vi "1296_usbUart.vi"(0 "VISA resource name":refnum<visa-resource-name>, 5 "command":string, 7 "r/w":enum16{"read", "write"}(ring), 9 "resetValues":bool, 11 "error in (no error)":errorcluster) -> (4 "byte Array":string[](array[string]), 6 "byte[4]":string, 8 "byte[5]":string, 15 "error out":errorcluster)   [LabVIEW 2018]
uses:
  <vilib>/Instr/_visa.llb/VISA Flush IO Buffer Mask.ctl
  <vilib>/Instr/_visa.llb/VISA Configure Serial Port (Instr).vi
panel:
  out "write buffer":string
  out "binary[7]":string
  out "number[7]":u32
  out "byte[7]":string
  out "number[4]":u32
  out "number[5]":u32
  out "number[6]":u32
  out "binary[6]":string
  out "byte[6]":string
  out "binary[5]":string
  out "binary[4]":string
  out "binary[3]":string
  out "number[3]":u32
  out "byte[3]":string
  out "number[0]":u32
  out "number[1]":u32
  out "number[2]":u32
  out "binary[2]":string
  out "byte[2]":string
  out "binary[1]":string
  out "byte[1]":string
  out "byte[0]":string
  out "binary[0]":string
  out "valid byte":string
  out "bytes at port":u32
  out "byte count":u32
  out "read buffer":string
  # "1. set visa\n2. set r/w\n3. enter command:\naddress/command/and any data if writing.\nwrite example: 0900 0001\nread example: 0900"
  # "Read Packet:\t\t\t\t\t\t\t\t\t\t\t                                                                                                                                                                                                                                                                                                                                              Example for w/r of relay1:\t\t\t\t\t\t\t\t\t\t\t\t\t\t\nAddress\t0x01 - Speed\t0x02 - Distance\t0x03 - Resistance\t0x04 - Incline\t0x09 - Box Control\t\t\t\t\t\t                                                                                                                                                                                                                0x09\tRead relay1\t\t\t\t\t\t\t\t\t\t\t\t\t\nCommand\tcommand for each protocol above - to be determined\t\t\t\t\t\t\t\t\t\t                                                                                                                                                                                                                                                   0x00\t\t\t\t\t\t\t\t\t\t\t\t\t\t\nType\t0x03 - Read\t0x06 - Write\t\t\t\t\t\t\t\t\t                                                                                                                                                                                                                                                                                                                    0x03\t\t\t\t\t\t\t\t\t\t\t\t\t\t\nByte Count\t0x01 would = Two bytes of data\t\t\t\t\t\t\t\t\t\t                                                                                                                                                                                                                                                                                          0x02\t\t\t\t\t\t\t\t\t\t\t\t\t\t\nEnd Charactors\t0x0D0A\t\t\t\t\t\t\t\t\t\t                                                                                                                                                                                                                                                                                                                             0x0D0A\t\t\t\t\t\t\t\t\t\t\t\t\t\t\n\t\t\t\t\t\t\t\t\t\t\t\t\t\t\t\t\t\t\t\t\t\t\t\t\t\n\t\t\t\t\t\t\t\t\t\t\t\t\t\t\t\t\t\t\t\t\t\t\t\t\t\n\t\t\t\t\t\t\t\t\t\t\t\t\t\t\t\t\t\t\t\t\t\t\t\t\t\nWrite Packet:\t\t\t\t\t\t\t\t\t\t\t\t\t\t\t\t\t\t\t\t\t\t\t\t\t\nAddress\t0x01 - Speed\t0x02 - Distance\t0x03 - Resistance\t0x04 - Incline\t0x09 - Box Control\t\t\t\t\t\t                                                                                                                                                                                                               0x09\tWrite relay1 on\t\t\t\t\t\t\t\t\t\t\t\t\t\nCommand\tcommand for each protocol above - to be determined\t\t\t\t\t\t\t\t\t\t                                                                                                                                                                                                                                                  0x00\t\t\t\t\t\t\t\t\t\t\t\t\t\t\nType\t0x03 - Read\t0x06 - Write\t\t\t\t\t\t\t\t\t                                                                                                                                                                                                                                                                                                                   0x06\t\t\t\t\t\t\t\t\t\t\t\t\t\t\nByte Count\t0x01 would = Two bytes of data\t\t\t\t\t\t\t\t\t\t                                                                                                                                                                                                                                                                                         0x02\t\t\t\t\t\t\t\t\t\t\t\t\t\t\nData\tEach data piece will be 2 bytes.\t\t\t\t\t\t\t\t\t                                                                                                                                                                                                                                                                                                      \t0x0001\t\t\t\t\t\t\t\t\t\t\t\t\t\t\nEnd Charactors\t0x0D0A\t\t\t\t\t\t\t\t\t\t                                                                                                                                                                                                                                                                                                                            0x0D0A\t\t\t\t\t\t\t\t\t\t\t\t\t\t\n\t\t\t\t\t\t\t\t\t\t\t\t\t\t\t\t\t\t\t\t\t\t\t\t\t\nResponses will match on address, command, type, and byte count as what was sent.\t\t\t\t\t\t\t\t\t\t\t\t\t\t\t\t\t\t\t\t\t\t\t\t\t\n\t\t\t\t\t\t\t\t\t\t\t\t\t\t\t\t\t\t\t\t\t\t\t\t\t\nResponse Read Packet:\t\t\t\t\t\t\t\t\t\t\t\t\t\t\t\t\t\t\t\t\t\t\t\t\t\n\t\t\t\t\t\t\t\t\t\t\t\t\t\t\t\t\t\t\t\t\t\t\t\t\t\nAddress\t0x01\tIncline\t\t\t\t\t\t\t\t\t                                                                                                                                                                                                                                                                                                                                  0x09\t\t\t\t\t\t\t\t\t\t\t\t\t\t\nCommand\t0x04\tCommand 4 (maybe Read incline)\t\t\t\t\t\t\t\t\t                                                                                                                                                                                                                                                                             0x00\t\t\t\t\t\t\t\t\t\t\t\t\t\t\nType\t0x03\t\t\t\t\t\t\t\t\t                                                                                                                                                                                                                                                                                                                                                   \t0x06\t\t\t\t\t\t\t\t\t\t\t\t\t\t\nByte Count\t0x02\tRead 2 bytes\t\t\t\t\t\t\t\t\t                                                                                                                                                                                                                                                                                                                  0x02\t\t\t\t\t\t\t\t\t\t\t\t\t\t\nData\t0x0000A\tRead incline\tEach data packet will be 16 bit, 2 bytes.  Mainly because I'll have to make an array for these so they will all be the same size.\t\t\t\t\t\t\t\t                                                                                                 0x0001\t\t\t\t\t\t\t\t\t\t\t\t\t\t\nData...\t0x0005\tNext byte, maybe read sense count?\t\t\t\t\t\t\t\t\t                                                                                                                                                                                                                                                                             0x000A\t\t\t\t\t\t\t\t\t\t\t\t\t\t\nEnd Characters\t0x0D0A\t\t\t\t\t\t\t\t\t\t                                                                                                                                                                                                                                                                                                                            0x0D0A\t\t\t\t\t\t\t\t\t\t\t\t\t\t\n\t\t\t\t\t\t\t\t\t\t\t\t\t\t\t\t\t\t\t\t\t\t\t\t\t\nResponse Write Packet :\t\t\t\t\t\t\t\t\t\t\t\t\t\t\t\t\t\t\t\t\t\t\t\t\t\nAddress\t0x0A\t\t\t\t\t\t\t\t\t\t                                                                                                                                                                                                                                                                                                                                             0x09\t\t\t\t\t\t\t\t\t\t\t\t\t\t\nCommand\t0x01\t\t\t\t\t\t\t\t\t\t                                                                                                                                                                                                                                                                                                                                        0x00\t\t\t\t\t\t\t\t\t\t\t\t\t\t\nType\t0x06\t\t\t\t\t\t\t\t\t\t                                                                                                                                                                                                                                                                                                                                                   0x06\t\t\t\t\t\t\t\t\t\t\t\t\t\t\nByte Count\t0x03\t\t\t\t\t\t\t\t\t\t                                                                                                                                                                                                                                                                                                                                       0x02\t\t\t\t\t\t\t\t\t\t\t\t\t\t\nEnd Charactors\t0x0D0A\t\t\t\t\t\t\t\t\t\t                                                                                                                                                                                                                                                                                                                           0x0D0A\t\t\t\t\t\t\t\t\t\t\t\t\t\t\n\t\t\t\t\t\t\t\t\t\t\t\t\t\t\t\t\t\t\t\t\t\t\t\t\t\nError Responses:\tAddress response is 0xFF then a code below\t\t\t\t\t\t\t\t\t\t\t\t\t\t\t\t\t\t\t\t\t\t\t\t\nBad End Charactors\t0x01\tMissing 0x0D0A at end of communication word\t\t\t\t\t\t\t\t\t\t\t\t\t\t\t\t\t\t\t\t\t\t\t\nRead bytes over run\t0x02\t\t\t\t\t\t\t\t\t\t\t\t\t\t\t\t\t\t\t\t\t\t\t\t\nWrite bytes over run\t0x03\t\t\t\t\t\t\t\t\t\t\t\t\t\t\t\t\t\t\t\t\t\t\t\t\nInvalid Address\t0x04\t\t\t\t\t\t\t\t\t\t\t\t\t\t\t\t\t\t\t\t\t\t\t\t\nInvalid Command\t0x05\t\t\t\t\t\t\t\t\t\t\t\t\t\t\t\t\t\t\t\t\t\t\t\t\nR/W Command Failed\t0x06\tRead / Write to device failed\t\t\t\t\t\t\t\t\t\t\t\t\t\t\t\t\t\t\t\t\t\t\t\n\t\t\t\t\t\t\t\t\t\t\t\t\t\t\t\t\t\t\t\t\t\t\t\t\t\n\t\t\t\t\t\t\t\t\t\t\t\t\t\t\t\t\t\t\t\t\t\t\t\t\t\n\t\t\t\t\t\t\t\t\t\t\t\t\t\t\t\t\t\t\t\t\t\t\t\t\t\nNOTE:  All commands can be read from or written to.  Commands not marked as writable, should not be written to.  Results are could cause servere confustion or damage."
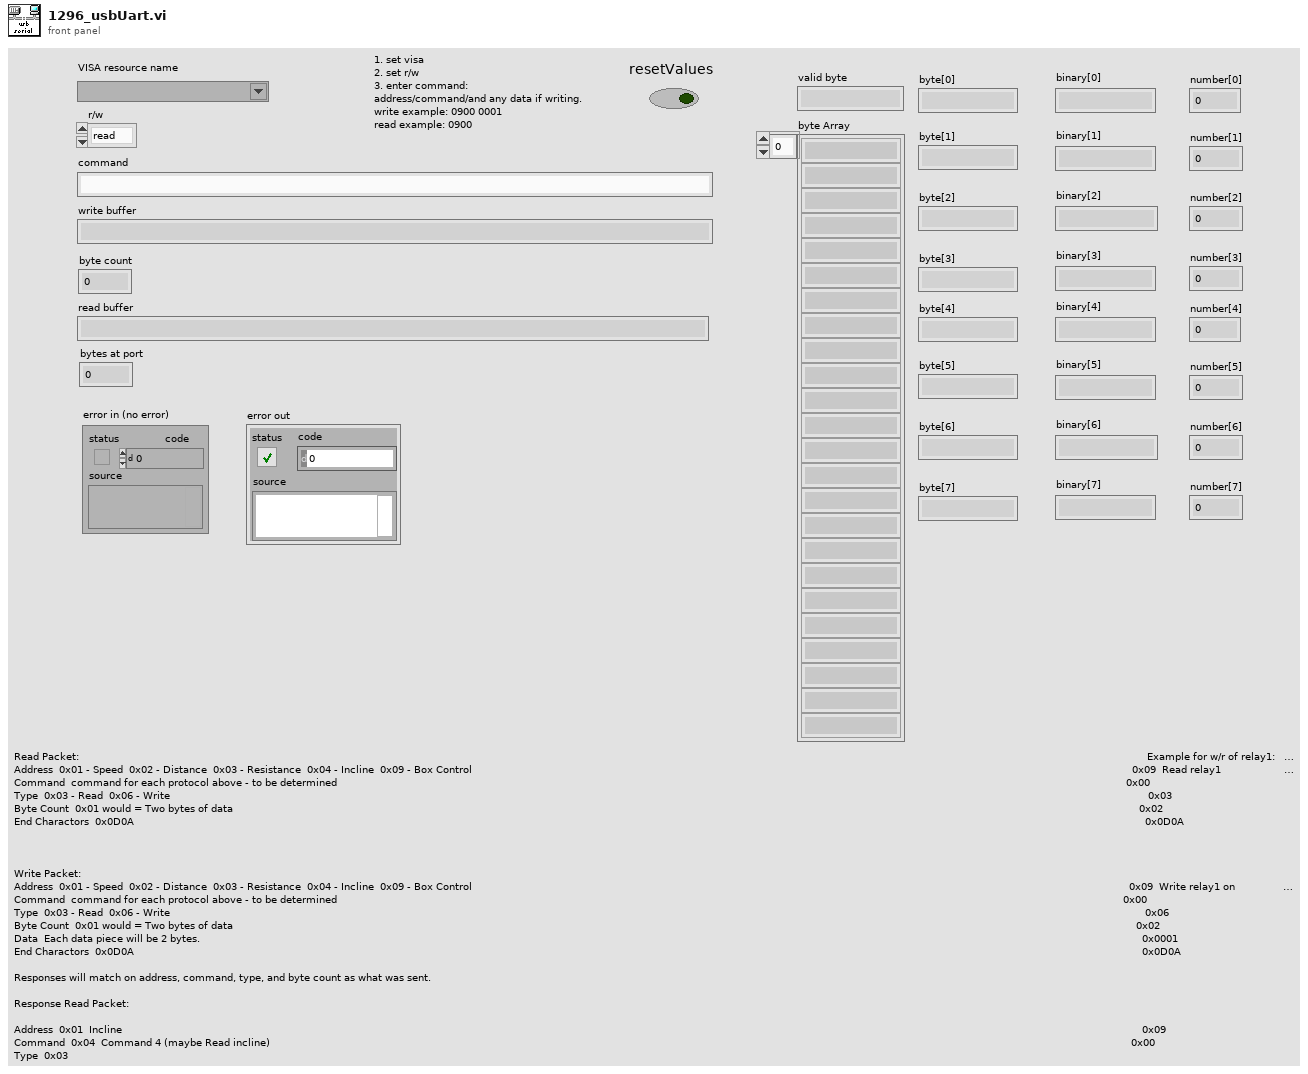
[diagram p1: front panel]
types:
  T1 = typedef "VISA Flush IO Buffer Mask.ctl" = u16
  T2 = cluster{"[0]":string, "[1]":string, "[2]":string, "[3]":string, "[4]":string, "[5]":string, "[6]":string, "[7]":string, "[8]":string}
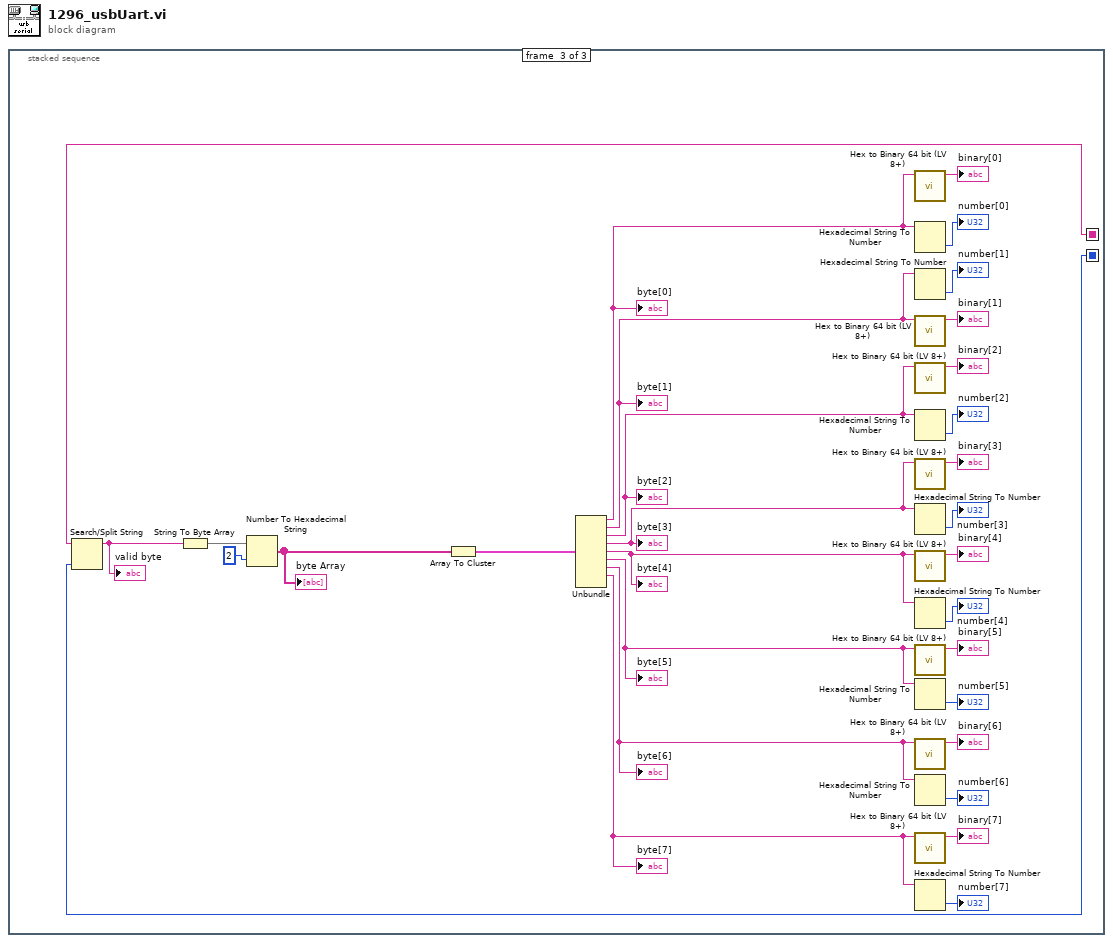
[diagram p0: block diagram]
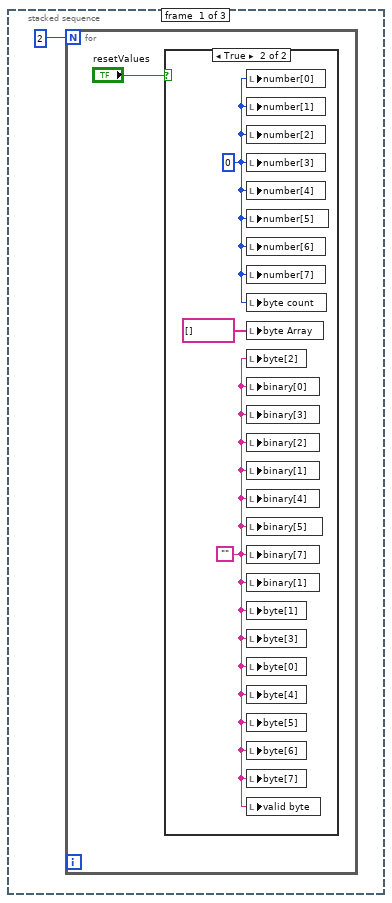
[diagram p2: hidden frame]
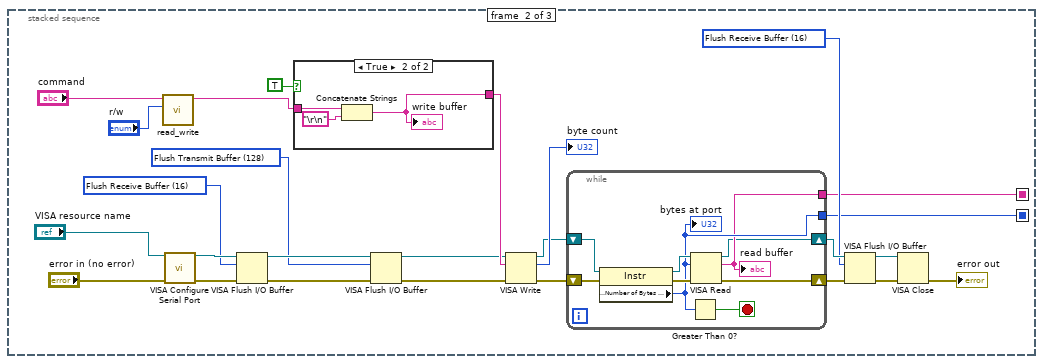
[diagram p4: hidden frame]
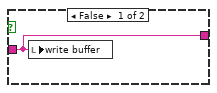
[diagram p5: hidden frame]
diagram:
  n1 = stacked-sequence {
    seq-local: [_ w10 _] -> [_ _ w46]
    seq-local: [_ w9 _] -> [_ _ w45]
    frame #0 {
      n2 = for {
        N: 2 -> [_]
        n3 = case shown="True" "resetValues" {
          frame False {
          }
          frame True {
            w4 = u32 0
            w3 = ""
            n4 = local write "number[0]"(w4) -> ()
            n5 = local write "number[1]"(w4) -> ()
            n6 = local write "number[2]"(w4) -> ()
            n7 = local write "number[3]"(w4) -> ()
            n8 = local write "number[4]"(w4) -> ()
            n9 = local write "number[5]"(w4) -> ()
            n10 = local write "number[6]"(w4) -> ()
            n11 = local write "number[7]"(w4) -> ()
            n12 = local write "byte count"(w4) -> ()
            n13 = local write "byte Array"(string[] []) -> ()
            n14 = local write "byte[2]"(w3) -> ()
            n15 = local write "binary[0]"(w3) -> ()
            n16 = local write "binary[3]"(w3) -> ()
            n17 = local write "binary[2]"(w3) -> ()
            n18 = local write "binary[1]"(w3) -> ()
            n19 = local write "binary[4]"(w3) -> ()
            n20 = local write "binary[5]"(w3) -> ()
            n21 = local write "binary[7]"(w3) -> ()
            n22 = local write "binary[1]"(w3) -> ()
            n23 = local write "byte[1]"(w3) -> ()
            n24 = local write "byte[3]"(w3) -> ()
            n25 = local write "byte[0]"(w3) -> ()
            n26 = local write "byte[4]"(w3) -> ()
            n27 = local write "byte[5]"(w3) -> ()
            n28 = local write "byte[6]"(w3) -> ()
            n29 = local write "byte[7]"(w3) -> ()
            n30 = local write "valid byte"(w3) -> ()
          }
        }
      }
    }
    frame #1 {
      w14 = T1 128 items=["Flush Receive Buffer"=16, "Write Transmit Buffer to Device"=32, "Flush Receive Buffer (No I/O)"=64, "Flush Transmit Buffer"=128] ("Mask")
      w13 = T1 16 items=["Flush Receive Buffer"=16, "Write Transmit Buffer to Device"=32, "Flush Receive Buffer (No I/O)"=64, "Flush Transmit Buffer"=128] ("Mask")
      w12 = T1 16 items=["Flush Receive Buffer"=16, "Write Transmit Buffer to Device"=32, "Flush Receive Buffer (No I/O)"=64, "Flush Transmit Buffer"=128] ("Mask")
      n31 = call "read_write.vi"("Enum"="r/w", "command_in"="command") -> ("command_out"=w8:string)  [unwired: 9 in]
      n32 = call-poly "VISA Configure Serial Port"("VISA resource name"="VISA resource name", "error in (no error)"="error in (no error)") -> ("VISA resource name out"=w19:refnum<visa-resource-name>, "error out"=w20:errorcluster)  [unwired: 12 in]
      n33 = VISA Flush I/O Buffer(VISA resource name=w19, mask (16)=w13, error in (no error)=w20) -> (VISA resource name out=w23:refnum<visa-resource-name>, error out=w22:errorcluster)
      n34 = case shown="True" TRUE ("Add 0D0A") {
        tunnel: w8 -> [w32 w34]
        tunnel: [w32 w33] -> w29
        frame False {
          n35 = local write "write buffer"(w32) -> ()
        }
        frame True {
          n36 = Concatenate Strings(w34, "\r\n") -> (w33:string)
          "write buffer" <- w33
        }
      }
      n37 = VISA Flush I/O Buffer(VISA resource name=w23, mask (16)=w14, error in (no error)=w22) -> (VISA resource name out=w24:refnum<visa-resource-name>, error out=w25:errorcluster)
      n38 = VISA Write(VISA resource name=w24, write buffer=w29, error in (no error)=w25) -> (VISA resource name out=w15:refnum<visa-resource-name>, return count=→"byte count":u32, error out=w16:errorcluster)
      n39 = while {
        tunnel: [w38] -> w10
        tunnel: [w39] -> w9
        shift-right: [w36] -> w21
        shift-left: w15 -> [w44]
        shift-right: [w37] -> w18
        shift-left: w16 -> [w43]
        stop <- w40 stop-if-true
        n40 = property class="Instr"(reference=w44, error in=w43) -> (reference out=w41:refnum<visa-resource-name>, error out=w42:errorcluster, "Serial Settings:Number of Bytes at Serial Port"=w39:u32)
        "bytes at port" <- w39
        n41 = Greater Than 0?(x=w39) -> (x > 0?=w40:bool)
        n42 = VISA Read(VISA resource name=w41, byte count=w39, error in (no error)=w42) -> (VISA resource name out=w36:refnum<visa-resource-name>, read buffer=w38:string, error out=w37:errorcluster)  [unwired: 1 out]
        "read buffer" <- w38
      }
      n43 = VISA Flush I/O Buffer(VISA resource name=w21, mask (16)=w12, error in (no error)=w18) -> (VISA resource name out=w26:refnum<visa-resource-name>, error out=w27:errorcluster)
      n44 = VISA Close(VISA resource name=w26, error in (no error)=w27) -> (error out=→"error out":errorcluster)
    }
    frame #2 {
      n45 = Search/Split String(string=w46, offset (0)=w45) -> (substring before match=w49:string)  [unwired: 1 in, 2 out]
      "valid byte" <- w49
      n46 = String To Byte Array(string=w49) -> (unsigned byte array=w48:u8[])
      n47 = Number To Hexadecimal String(1:i16 2 ("width (-)"), 2:w48) -> (0:w75:string[])
      "byte Array" <- w75
      n48 = Array To Cluster(array=w75) -> (cluster=w60:T2)
      n49 = Unbundle(w60) -> ("[0]"=w59:string, "[1]"=w58:string, "[2]"=w52:string, "[3]"=w62:string, "[4]"=w67:string, "[5]"=w68:string, "[6]"=w69:string, "[7]"=w70:string)  [unwired: 1 out]
      "byte[0]" <- w59
      "byte[1]" <- w58
      "byte[2]" <- w52
      "byte[3]" <- w62
      "byte[4]" <- w67
      "byte[5]" <- w68
      "byte[6]" <- w69
      "byte[7]" <- w70
      n50 = call "Hex to Binary 64 bit (LV 8+).vi"("Hexadecimal String"=w59) -> ("Binary String"=→"binary[0]":string)  [unwired: 6 in, 2 out]
      n51 = Hexadecimal String To Number(string=w59) -> (number=→"number[0]":u32)  [unwired: 2 in, 1 out]
      n52 = Hexadecimal String To Number(string=w58) -> (number=→"number[1]":u32)  [unwired: 2 in, 1 out]
      n53 = call "Hex to Binary 64 bit (LV 8+).vi"("Hexadecimal String"=w58) -> ("Binary String"=→"binary[1]":string)  [unwired: 6 in, 2 out]
      n54 = call "Hex to Binary 64 bit (LV 8+).vi"("Hexadecimal String"=w52) -> ("Binary String"=→"binary[2]":string)  [unwired: 6 in, 2 out]
      n55 = Hexadecimal String To Number(string=w52) -> (number=→"number[2]":u32)  [unwired: 2 in, 1 out]
      n56 = call "Hex to Binary 64 bit (LV 8+).vi"("Hexadecimal String"=w62) -> ("Binary String"=→"binary[3]":string)  [unwired: 6 in, 2 out]
      n57 = Hexadecimal String To Number(string=w62) -> (number=→"number[3]":u32)  [unwired: 2 in, 1 out]
      n58 = call "Hex to Binary 64 bit (LV 8+).vi"("Hexadecimal String"=w67) -> ("Binary String"=→"binary[4]":string)  [unwired: 6 in, 2 out]
      n59 = Hexadecimal String To Number(string=w67) -> (number=→"number[4]":u32)  [unwired: 2 in, 1 out]
      n60 = call "Hex to Binary 64 bit (LV 8+).vi"("Hexadecimal String"=w68) -> ("Binary String"=→"binary[5]":string)  [unwired: 6 in, 2 out]
      n61 = Hexadecimal String To Number(string=w68) -> (number=→"number[5]":u32)  [unwired: 2 in, 1 out]
      n62 = call "Hex to Binary 64 bit (LV 8+).vi"("Hexadecimal String"=w69) -> ("Binary String"=→"binary[6]":string)  [unwired: 6 in, 2 out]
      n63 = Hexadecimal String To Number(string=w69) -> (number=→"number[6]":u32)  [unwired: 2 in, 1 out]
      n64 = call "Hex to Binary 64 bit (LV 8+).vi"("Hexadecimal String"=w70) -> ("Binary String"=→"binary[7]":string)  [unwired: 6 in, 2 out]
      n65 = Hexadecimal String To Number(string=w70) -> (number=→"number[7]":u32)  [unwired: 2 in, 1 out]
    }
  }
